vi "Test Sequence in XML.vi"(7 "Command":T2, 8 "error in (no error)":errorcluster, 11 "Test Seletor":string) -> (0 "error out":errorcluster, 3 "Test Description":T1)   [LabVIEW 2021, in "User Interface.lvlib"]
uses:
  User Interface.lvlib
  Test Squence Command.ctl
  Test Description.ctl
  Create Path Command.ctl
  <vilib>/Utility/xml.llb/Write to XML File(string).vi
  <vilib>/Utility/xml.llb/Read From XML File(array).vi
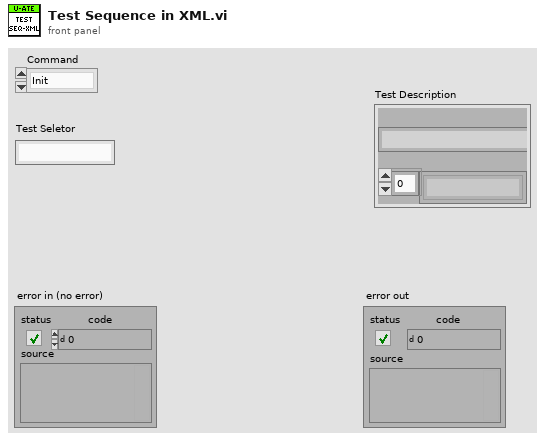
[diagram p1: front panel]
types:
  T1 = typedef "User Interface.lvlib/Test Description.ctl" = cluster{"Test Name":string, "Test Step":string[]}
  T2 = typedef "User Interface.lvlib/Test Squence Command.ctl" = enum16{"Init", "Read", "Close"}
  T3 = typedef "User Interface.lvlib/Create Path Command.ctl" = enum16{"Authentication", "Hardware", "Configuration", "Calibration", "Instrument", "Test Description", "Serial Data", "ARINC Data", "CAN Data", "Data", "Report", "Action log", "Error Log"}
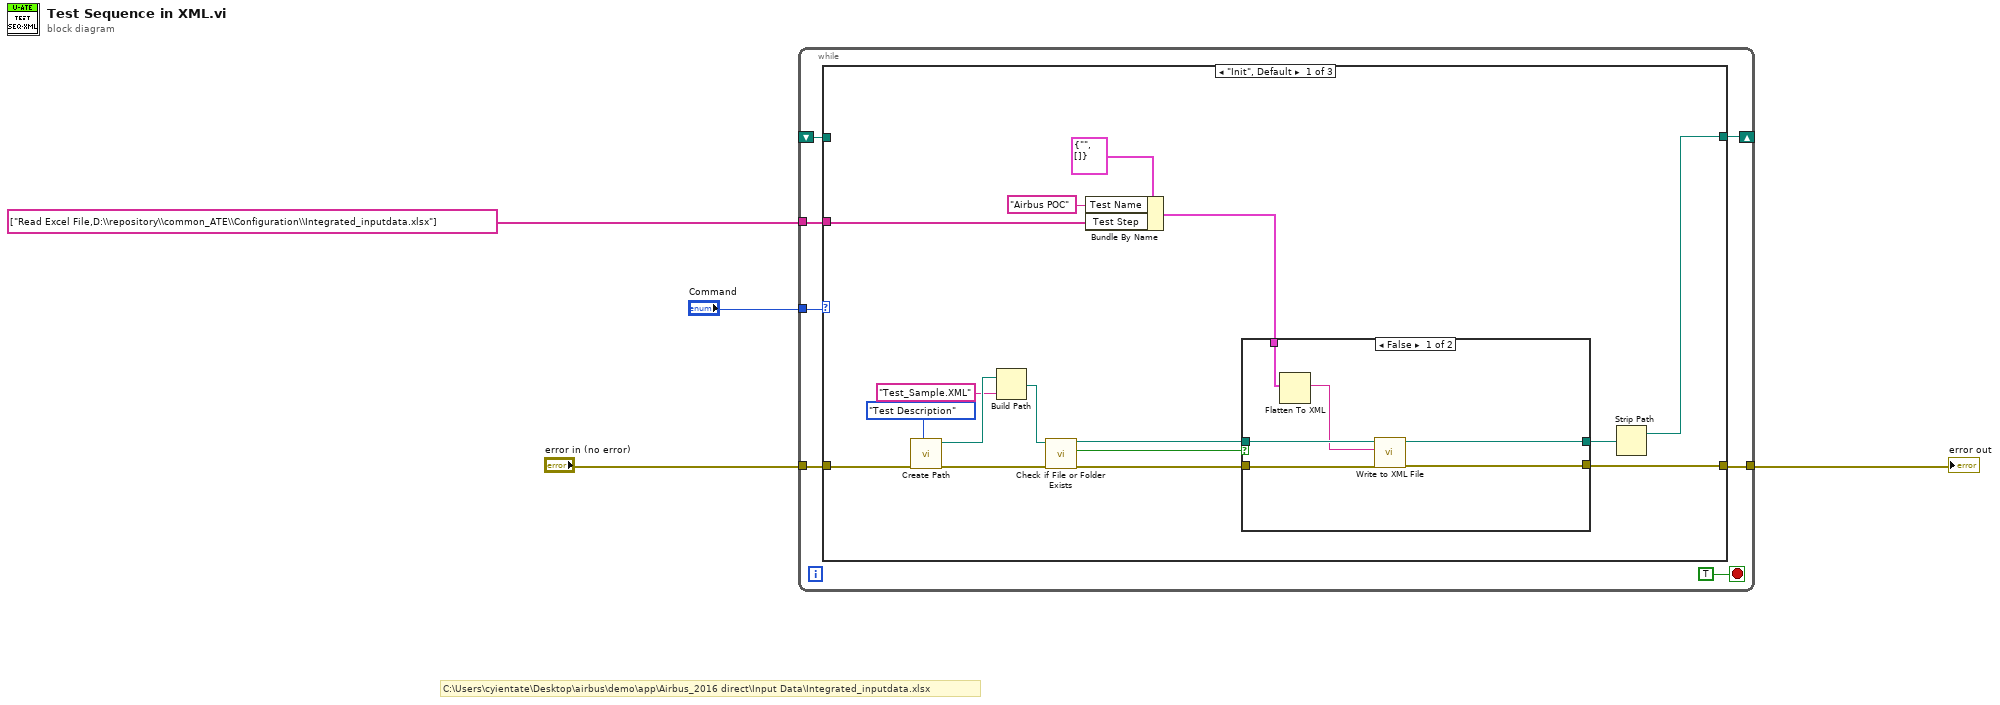
[diagram p0: block diagram]
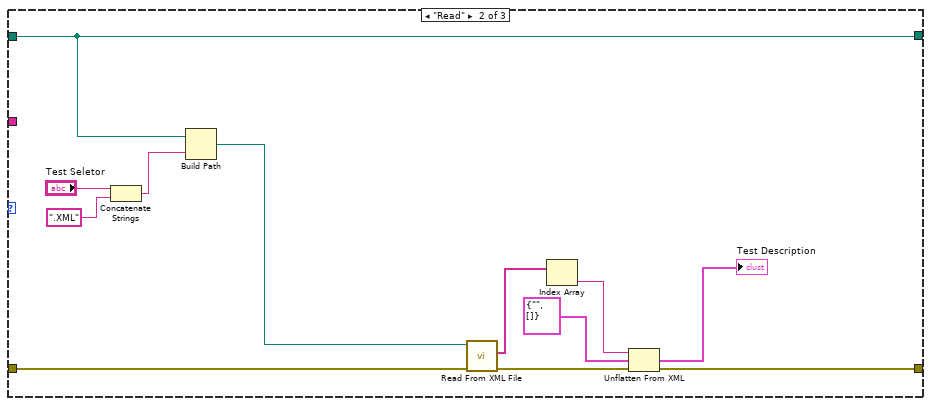
[diagram p3: hidden frame]
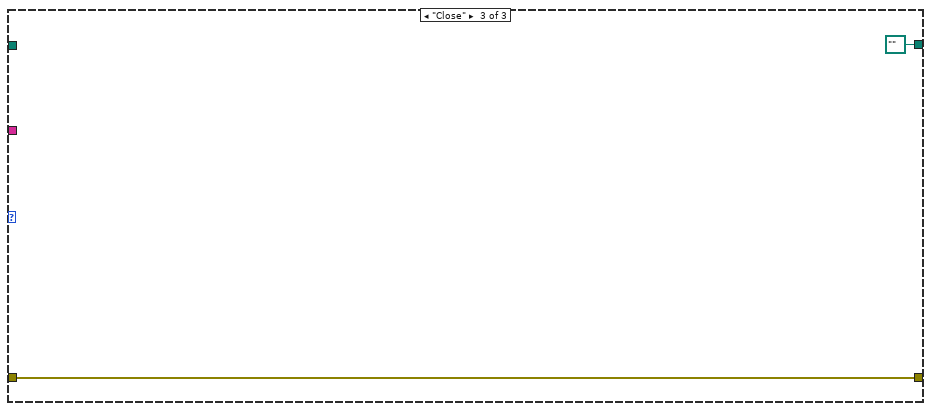
[diagram p4: hidden frame]
diagram:
  # "C:\\Users\\cyientate\\Desktop\\airbus\\demo\\app\\Airbus_2016 direct\\Input Data\\Integrated_inputdata.xlsx"
  n1 = while {
    tunnel: "error in (no error)" -> [w9]
    tunnel: "Command" -> [w10]
    tunnel: [w8] -> w2
    shift-right: [w7] -> _
    shift-left: _ -> [w6]
    tunnel: string[] ["Read Excel File,D:\\repository\\common_ATE\\Configuration\\Integrated_inputdata.xlsx"] -> [w5]
    stop <- TRUE stop-if-true
    n2 = case shown="\"Init\", Default" w10 {
      tunnel: w9 -> [w27 w43 w49]
      tunnel: [w19 w37 w49] -> w8
      tunnel: [w16 w44 path "" ("stripped path")] -> w7
      tunnel: w6 -> [_ w44 _]
      tunnel: w5 -> [w12 _ _]
      frame "Init", Default {
        n3 = call "Create Path.vi"("Path Command"=Create_Path_Command."Test Description", "error in (no error)"=w27) -> ("error out"=w26:errorcluster, "created path"=w24:path)  [unwired: 8 in]
        n4 = Build Path(base path=w24, name or relative path="Test_Sample.XML") -> (appended path=w22:path)
        n5 = call <vilib>:"Check if File or Folder Exists.vi"("error in (no error)"=w26, "path"=w22) -> ("error out"=w21:errorcluster, "file or folder exists?"=w20:bool, "dup path"=w18:path)  [unwired: 7 in]
        n6 = Bundle By Name(cluster=T1 {"Test Name"="", "Test Step"=[]}, "Test Name"="Airbus POC", "Test Step"=w12) -> (w14:T1)
        n7 = case shown="False" w20 {
          tunnel: w21 -> [w33 w34]
          tunnel: [w32 w34] -> w19
          tunnel: w18 -> [w31 w35]
          tunnel: [w29 w35] -> w17
          tunnel: w14 -> [w28 _]
          frame False {
            n8 = Flatten To XML(6:w28) -> (2:w30:string)
            n9 = call-poly <vilib>:"Write to XML File.vi"("error in (no error)"=w33, "XML Input"=w30, "XML File Path"=w31) -> ("error out"=w32:errorcluster, "XML File Path(duplicate)"=w29:path)  [unwired: 6 in, 1 out]
          }
          frame True {
          }
        }
        n10 = Strip Path(path=w17) -> (stripped path=w16:path)  [unwired: 1 out]
      }
      frame "Read" {
        n11 = Concatenate Strings("Test Seletor", ".XML" ("string")) -> (w45:string)
        n12 = Build Path(base path=w44, name or relative path=w45) -> (appended path=w42:path)
        n13 = call-poly <vilib>:"Read From XML File.vi"("error in (no error)"=w43, "XML File Path"=w42) -> ("error out"=w38:errorcluster, "XML Elements"=w41:string[])  [unwired: 7 in, 1 out]
        n14 = Index Array(array=w41) -> (element=w40:string)  [unwired: 1 in]
        n15 = Unflatten From XML(xml string=w40, type=T1 {"Test Name"="", "Test Step"=[]}, error in (no error)=w38) -> (value=→"Test Description":T1, error out=w37:errorcluster)
      }
      frame "Close" {
      }
    }
  }
  "error out" <- w2
